vi "configuration_rm_vlc.vi"() -> (3 "configuration_rm_vlc":T1)   [LabVIEW 2023]
panel:
  in  "configuration_rm_vlc":T1={"chunk"=4096, "mode"=1, "divisor"=1, "profile"=3, "level"=255, "bitrate"=0, "options_size"=-1, "options_data"=0, "_reserved_0"=0}
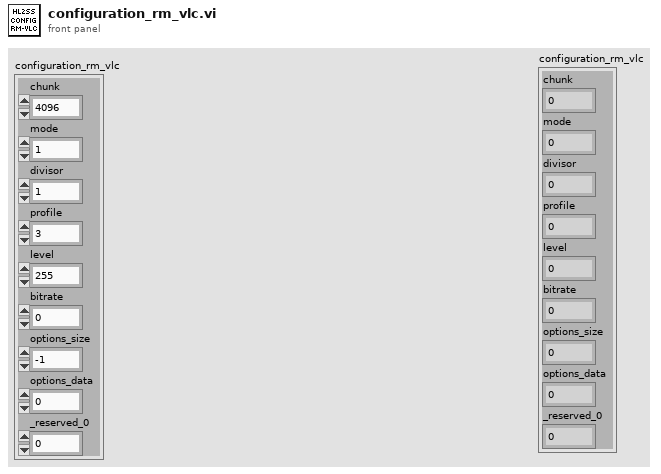
[diagram p1: front panel]
types:
  T1 = cluster{"chunk":u64, "mode":u8, "divisor":u8, "profile":u8, "level":u8, "bitrate":u32, "options_size":i64, "options_data":u64, "_reserved_0":u64}
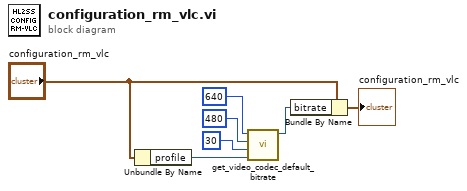
[diagram p0: block diagram]
diagram:
  n1 = Unbundle By Name("configuration_rm_vlc") -> ("profile"=w2:u8)
  n2 = call "get_video_codec_default_bitrate.vi"("profile"=w2, "framerate"=u8 30, "height"=u16 480, "width"=u16 640) -> ("bitrate"=w4:u32)  [unwired: 7 in]
  n3 = Bundle By Name(cluster="configuration_rm_vlc", "bitrate"=w4) -> (→"configuration_rm_vlc":T1)
